vi "Add Points Int.vi"(7 "rebuild_threshold":sgl=1.0, 8 "error in (no error)":errorcluster, 10 "points":i32[][](array[numeric]), 11 "KD Tree Int in":refnum<class "KD Tree Int.lvclass">) -> (0 "error out":errorcluster, 3 "KD Tree Int out":refnum<class "KD Tree Int.lvclass">)   [LabVIEW 2020, in "KD Tree.lvlib" / "KD Tree Int.lvclass"]
uses:
  KD Tree Int.lvclass
  KD Tree.lvlib
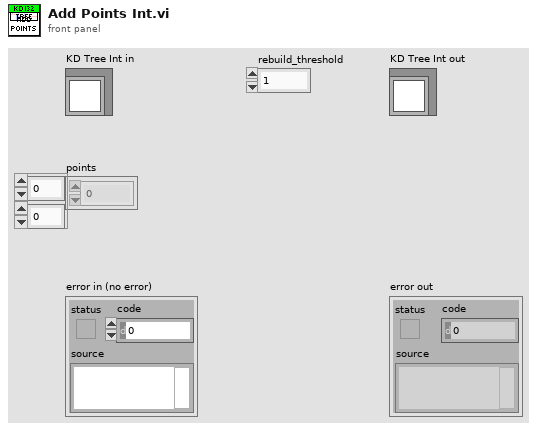
[diagram p1: front panel]
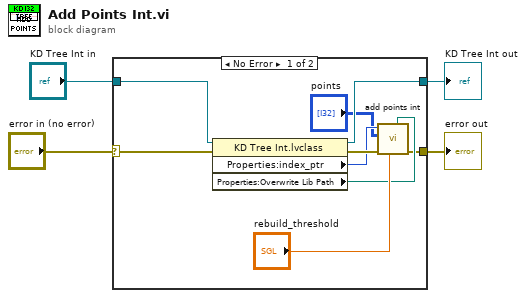
[diagram p0: block diagram]
diagram:
  n1 = case shown="No Error" "error in (no error)" {
    selector: "error in (no error)" -> [w13 w15]
    tunnel: [w5 w15] -> w3
    tunnel: [w10 w14] -> w1
    tunnel: "KD Tree Int in" -> [w11 w14]
    frame No Error {
      n2 = property class="KD Tree Int.lvclass"(reference=w11, error in=w13) -> (reference out=w10:refnum<class "KD Tree Int.lvclass">, error out=w12:errorcluster, "Properties:index_ptr"=w9:u64, "Properties:Overwrite Lib Path"=w6:path)
      n3 = call "add points int.vi"("Overwrite Lib Path"=w6, "rebuild_threshold"="rebuild_threshold", "error in (no error)"=w12, "points"="points", "index_ptr"=w9) -> ("error out"=w5:errorcluster)  [unwired: 5 in, 1 out]
    }
    frame Error {
    }
  }
  "error out" <- w3
  "KD Tree Int out" <- w1
